vi "Generate Filenames_atw.vi"(11 "path":path) -> (0 "TDMS Path":path, 1 "Dalsa Path":path, 2 "Basler Path":path, 3 "WebCam Path":path, 4 "Analog file name":string="F:\\Data\\130725_14_35_2625", 5 "CSV Path":path)   [LabVIEW 2013]
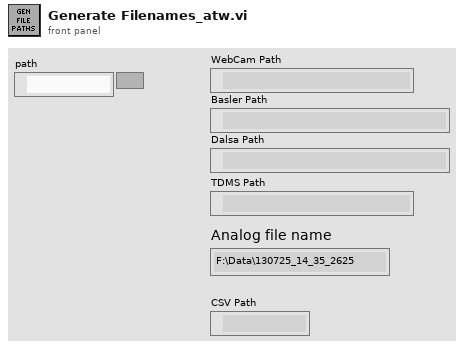
[diagram p1: front panel]
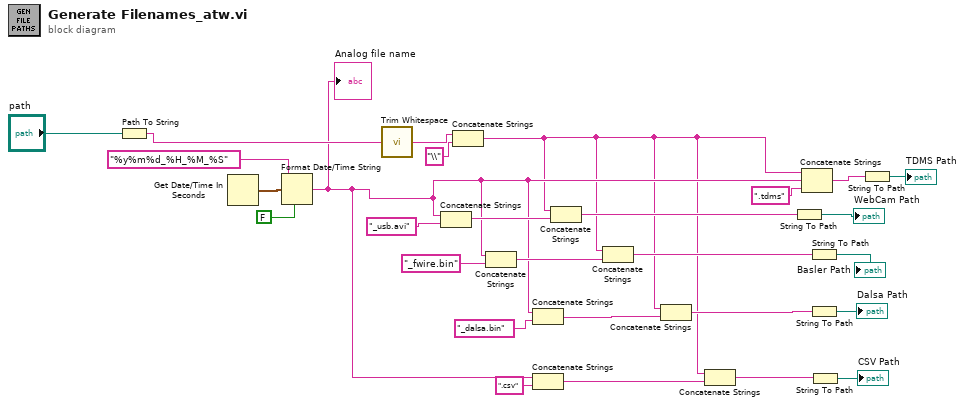
[diagram p0: block diagram]
diagram:
  n1 = Path To String(path="path") -> (string=w10:string)
  n2 = Get Date/Time In Seconds() -> (seconds since 1Jan1904=w27:timestamp)
  n3 = Format Date/Time String(time format string (%c)="%y%m%d_%H_%M_%S", seconds (now)=w27, UTC format=FALSE) -> (date/time string=w6:string)
  "Analog file name" <- w6
  n4 = call <vilib>:"Trim Whitespace.vi"("string"=w10) -> ("trimmed string"=w8:string)  [unwired: 1 in]
  n5 = Concatenate Strings(w6, "_usb.avi") -> (w25:string)
  n6 = Concatenate Strings(w8, "\\" ("string")) -> (w3:string)
  n7 = Concatenate Strings(w6, "_fwire.bin" ("string")) -> (w19:string)
  n8 = Concatenate Strings(w6, "_dalsa.bin") -> (w23:string)
  n9 = Concatenate Strings(w6, ".csv" ("string")) -> (w4:string)
  n10 = Concatenate Strings(w3, w25) -> (w21:string)
  n11 = Concatenate Strings(w3, w19) -> (w18:string)
  n12 = Concatenate Strings(w3, w23) -> (w22:string)
  n13 = Concatenate Strings(w3, w4) -> (w2:string)
  n14 = String To Path(string=w21) -> (path=→"WebCam Path":path)
  n15 = Concatenate Strings(w3, w6, ".tdms" ("string")) -> (w11:string)
  n16 = String To Path(string=w18) -> (path=→"Basler Path":path)
  n17 = String To Path(string=w22) -> (path=→"Dalsa Path":path)
  n18 = String To Path(string=w2) -> (path=→"CSV Path":path)
  n19 = String To Path(string=w11) -> (path=→"TDMS Path":path)
